vi "Get Protocol.vi"(8 "error in (no error)":errorcluster, 11 "instrument addon refnum in":T1 format="%.0x") -> (0 "error out":errorcluster, 2 "protocol":refnum<class "Protocol Parent.lvclass">, 3 "instrument addon refnum out":T1=18446744073709551615 format="%.0x")   [LabVIEW 2020, in "Instrument Addon Scripting API.lvlib"]
doc: "Outputs a protocol object based on the specified Instrument Addon Custom Device. \n\nThe protocol is formatted as one of the following classes: TCP.lvclass, UDP.lvclass, VISA.lvclass, RS-xxx.lvclass, AK TCP.lvclass, AK RS-xxx.lvclass, RS-xxx to GPIB ConvBox.lvclass"
uses:
  Instrument Addon Scripting API.lvlib
  <vilib>/NI VeriStand/Custom Device API/Custom Device Item Ref.ctl
  Includes/Protocols.lvlibp/Protocol Parent/Protocol Parent.lvclass
  Addon/Addon Shared/Types/FG Control.ctl
  Includes/Protocols.lvlibp/RS-xxx/RS-xxx.lvclass
  C:/Users/nitest/Desktop/Git 2020/niveristand-instrument-addon-custom-device/Includes/Protocols.lvlibp/Protocol Parent/Protocol Parent.lvclass
  Includes/Protocols.lvlibp/AK RS-xxx/AK RS-xxx.lvclass
  C:/Users/nitest/Desktop/Git 2020/niveristand-instrument-addon-custom-device/Includes/Protocols.lvlibp/RS-xxx/RS-xxx.lvclass
  Includes/Protocols.lvlibp/VISA/VISA.lvclass
  Includes/Protocols.lvlibp/AK TCP/AK TCP.lvclass
  C:/Users/nitest/Desktop/Git 2020/niveristand-instrument-addon-custom-device/Includes/Protocols.lvlibp/TCP/TCP.lvclass
  Includes/Protocols.lvlibp/TCP/TCP.lvclass
  Includes/Protocols.lvlibp/UDP/UDP.lvclass
  Includes/Protocols.lvlibp/RS-xxx to GPIB ConvBox/RS-xxx to GPIB ConvBox.lvclass
  Addon/Addon Shared/SubVIs/Constants.vi
  <vilib>/NI/NI VeriStand Advanced SysDef API/SysDef API/SysDef.Property.Get.vi
  <vilib>/NI/NI VeriStand Advanced SysDef API/_SubVIs/SysDef.Property.Get.String.vi
  <vilib>/NI/NI VeriStand Advanced SysDef API/SysDef API/SysDef.Property.Set.vi
  <vilib>/NI/NI VeriStand Advanced SysDef API/_SubVIs/SysDef.Property.Set.String.vi
  <vilib>/Utility/LVClass/Get LV Class Default Value.vi
  <vilib>/NI VeriStand/Custom Device API/NI VeriStand - Get Item Property.vi
  <vilib>/NI VeriStand/Custom Device API/Get Item Property (String).vi
  <vilib>/NI VeriStand/Custom Device API/Get Item Property (U32).vi
  <vilib>/NI VeriStand/Custom Device API/Get Item Property (Boolean).vi
  <vilib>/NI VeriStand/Custom Device API/NI VeriStand - Set Item Property.vi
  <vilib>/NI VeriStand/Custom Device API/Set Item Property (String).vi
  <vilib>/NI VeriStand/Custom Device API/Set Item Property (U32).vi
  <vilib>/NI VeriStand/Custom Device API/Set Item Property (Boolean).vi
  Includes/Protocols.lvlibp/RS-xxx/Data Access/Write PortSettings.vi
  Includes/Protocols.lvlibp/VISA/Data Access/Write VISA Resource.vi
  Includes/Protocols.lvlibp/VISA/Data Access/Write Enable Termination Character.vi
  Includes/Protocols.lvlibp/VISA/Data Access/Write Termination Character.vi
  Includes/Protocols.lvlibp/VISA/Data Access/Write Timeout.vi
  Includes/Protocols.lvlibp/VISA/Data Access/Write Append Write Termination Character.vi
  Includes/Protocols.lvlibp/TCP/Data Access/Write IP Address.vi
  Includes/Protocols.lvlibp/TCP/Data Access/Write Port.vi
  Includes/Protocols.lvlibp/UDP/Data Access/Write Local IP Address.vi
  Includes/Protocols.lvlibp/UDP/Data Access/Write Local Port.vi
  Includes/Protocols.lvlibp/UDP/Data Access/Write Target IP Address.vi
  Includes/Protocols.lvlibp/UDP/Data Access/Write Target Port.vi
  Includes/Protocols.lvlibp/RS-xxx to GPIB ConvBox/Data Access/Write Port.vi
  Includes/Protocols.lvlibp/RS-xxx to GPIB ConvBox/Data Access/Write ConvBox Address.vi
  Includes/Protocols.lvlibp/RS-xxx to GPIB ConvBox/Data Access/Write Assert Ren with IFC.vi
  Includes/Protocols.lvlibp/RS-xxx to GPIB ConvBox/Data Access/Write System controller.vi
  Includes/Protocols.lvlibp/RS-xxx to GPIB ConvBox/Data Access/Write IST bit sense.vi
  Includes/Protocols.lvlibp/RS-xxx to GPIB ConvBox/Data Access/Write GPIB Address.vi
  Addon/Addon Shared/Instrument Addon Shared.lvlib
  <vilib>/NI VeriStand/Custom Device API/Custom Device API.lvlib
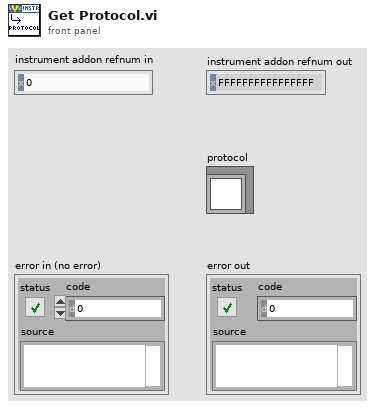
[diagram p1: front panel]
types:
  T1 = typedef "Custom Device API.lvlib/Custom Device Item Ref.ctl" = u64
  T2 = typedef "Instrument Addon Shared.lvlib/FG Control.ctl" = enum16{"Get", "Set"}
  T3 = cluster{"Port":string, "Baud Rate":u32, "Data Bits":u16, "Parity":enum16{"None", "Odd", "Even", "Mark", "Space"}, "Stop Bits":u16, "Flow Control":u16, "XON":enum16{"NUL", "SOH", "STX", "ETX", "EOT", "ENQ", "ACK", "BEL", "BS", "HT", "LF", "VT", "FF", "CR", "SO", "SI", "DLE", "DC1", "DC2", "DC3", "DC4", "NAK", "SYN", "ETB", "CAN", "EM", "SUB", "ESC", "FS", "GS", "RS", "US", "SP", "!", "\"", "#", "$", "%", "&", "'", "(", ")", "*", "+", ",", "- (-)", ".", "/", "0", "1", "2", "3", "4", "5", "6", "7", "8", "9", ":", ";", "<", "=", ">", "?", "@", "A", "B", "C", "D", "E", "F", "G", "H", "I", "J", "K", "L", "M", "N", "O", "P", "Q", "R", "S", "T", "U", "V", "W", "X", "Y", "Z", "[", "\\", "]", "^", "_", "`", "a", "b", "c", "d", "e", "f", "g", "h", "i", "j", "k", "l", "m", "n", "o", "p", "q", "r", "s", "t", "u", "v", "w", "x", "y", "z", "{", "|", "}", "~"}, "XOFF":enum16{"NUL", "SOH", "STX", "ETX", "EOT", "ENQ", "ACK", "BEL", "BS", "HT", "LF", "VT", "FF", "CR", "SO", "SI", "DLE", "DC1", "DC2", "DC3", "DC4", "NAK", "SYN", "ETB", "CAN", "EM", "SUB", "ESC", "FS", "GS", "RS", "US", "SP", "!", "\"", "#", "$", "%", "&", "'", "(", ")", "*", "+", ",", "- (-)", ".", "/", "0", "1", "2", "3", "4", "5", "6", "7", "8", "9", ":", ";", "<", "=", ">", "?", "@", "A", "B", "C", "D", "E", "F", "G", "H", "I", "J", "K", "L", "M", "N", "O", "P", "Q", "R", "S", "T", "U", "V", "W", "X", "Y", "Z", "[", "\\", "]", "^", "_", "`", "a", "b", "c", "d", "e", "f", "g", "h", "i", "j", "k", "l", "m", "n", "o", "p", "q", "r", "s", "t", "u", "v", "w", "x", "y", "z", "{", "|", "}", "~"}, "End Read on Termination Character":bool, "End Write on Termination Character":bool, "Termination Character":u8}
  T4 = typedef "Protocols.lvlibp/Protocol Parent.lvclass/Base Protocol Type.ctl" = enum16{"RS-XXX", "VISA", "TCPIP", "UDP", "GPIB ConvBox"}
  T5 = typedef "Instrument Addon Shared.lvlib/RSXXX Port Settings.ctl" = cluster{"Port":string, "Baud Rate":u32, "Data Bits":u16, "Parity":enum16{"None", "Odd", "Even", "Mark", "Space"}, "Stop Bits":u16, "Flow Control":u16, "XON":enum16{"NUL", "SOH", "STX", "ETX", "EOT", "ENQ", "ACK", "BEL", "BS", "HT", "LF", "VT", "FF", "CR", "SO", "SI", "DLE", "DC1", "DC2", "DC3", "DC4", "NAK", "SYN", "ETB", "CAN", "EM", "SUB", "ESC", "FS", "GS", "RS", "US", "SP", "!", "\"", "#", "$", "%", "&", "'", "(", ")", "*", "+", ",", "- (-)", ".", "/", "0", "1", "2", "3", "4", "5", "6", "7", "8", "9", ":", ";", "<", "=", ">", "?", "@", "A", "B", "C", "D", "E", "F", "G", "H", "I", "J", "K", "L", "M", "N", "O", "P", "Q", "R", "S", "T", "U", "V", "W", "X", "Y", "Z", "[", "\\", "]", "^", "_", "`", "a", "b", "c", "d", "e", "f", "g", "h", "i", "j", "k", "l", "m", "n", "o", "p", "q", "r", "s", "t", "u", "v", "w", "x", "y", "z", "{", "|", "}", "~"}, "XOFF":enum16{"NUL", "SOH", "STX", "ETX", "EOT", "ENQ", "ACK", "BEL", "BS", "HT", "LF", "VT", "FF", "CR", "SO", "SI", "DLE", "DC1", "DC2", "DC3", "DC4", "NAK", "SYN", "ETB", "CAN", "EM", "SUB", "ESC", "FS", "GS", "RS", "US", "SP", "!", "\"", "#", "$", "%", "&", "'", "(", ")", "*", "+", ",", "- (-)", ".", "/", "0", "1", "2", "3", "4", "5", "6", "7", "8", "9", ":", ";", "<", "=", ">", "?", "@", "A", "B", "C", "D", "E", "F", "G", "H", "I", "J", "K", "L", "M", "N", "O", "P", "Q", "R", "S", "T", "U", "V", "W", "X", "Y", "Z", "[", "\\", "]", "^", "_", "`", "a", "b", "c", "d", "e", "f", "g", "h", "i", "j", "k", "l", "m", "n", "o", "p", "q", "r", "s", "t", "u", "v", "w", "x", "y", "z", "{", "|", "}", "~"}, "End Read on Termination Character":bool, "End Write on Termination Character":bool, "Termination Character":u8}
  T6 = enum16{"NUL", "SOH", "STX", "ETX", "EOT", "ENQ", "ACK", "BEL", "BS", "HT", "LF", "VT", "FF", "CR", "SO", "SI", "DLE", "DC1", "DC2", "DC3", "DC4", "NAK", "SYN", "ETB", "CAN", "EM", "SUB", "ESC", "FS", "GS", "RS", "US", "SP", "!", "\"", "#", "$", "%", "&", "'", "(", ")", "*", "+", ",", "- (-)", ".", "/", "0", "1", "2", "3", "4", "5", "6", "7", "8", "9", ":", ";", "<", "=", ">", "?", "@", "A", "B", "C", "D", "E", "F", "G", "H", "I", "J", "K", "L", "M", "N", "O", "P", "Q", "R", "S", "T", "U", "V", "W", "X", "Y", "Z", "[", "\\", "]", "^", "_", "`", "a", "b", "c", "d", "e", "f", "g", "h", "i", "j", "k", "l", "m", "n", "o", "p", "q", "r", "s", "t", "u", "v", "w", "x", "y", "z", "{", "|", "}", "~"}
  T7 = typedef "Instrument Addon Shared.lvlib/VISA Settings.ctl" = cluster{"VISA Resource":string, "Enable Termination Character":bool, "Termination Character":u8, "Timeout":u32, "Append Write Termination Character":bool}
  T8 = typedef "Instrument Addon Shared.lvlib/TCPIP Settings.ctl" = cluster{"IP Address":string, "Port":u16}
  T9 = typedef "Instrument Addon Shared.lvlib/UDP Settings.ctl" = cluster{"Local IP Address":string, "Local Port":u16, "Target IP Address":string, "Target Port":u16}
  T10 = typedef "Instrument Addon Shared.lvlib/GPIB ConvBox Settings.ctl" = cluster{"Port":string, "ConvBox Address":string, "Assert Ren with IFC":bool, "System controller":bool, "IST bit sense":bool, "GPIB Address":string}
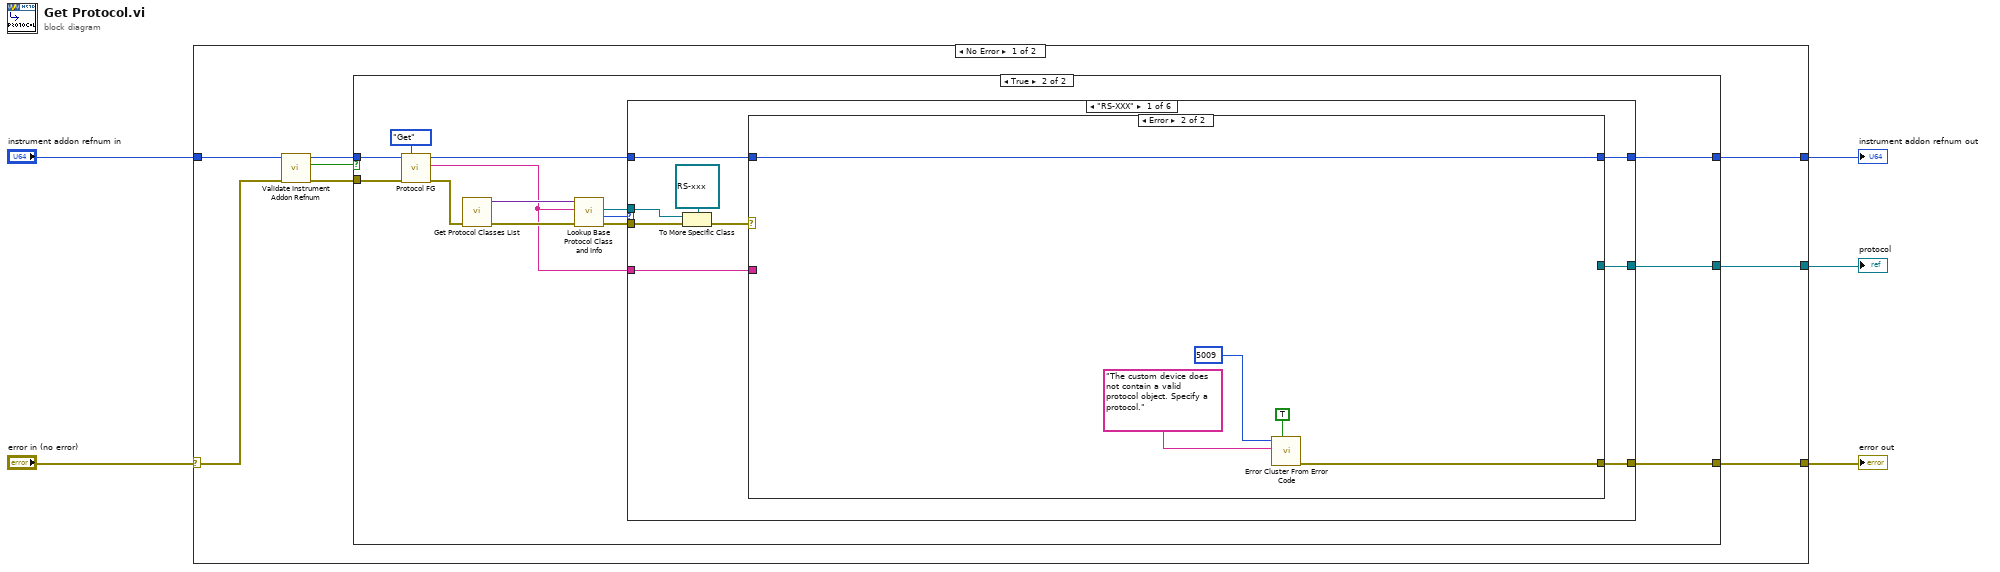
[diagram p0: block diagram]
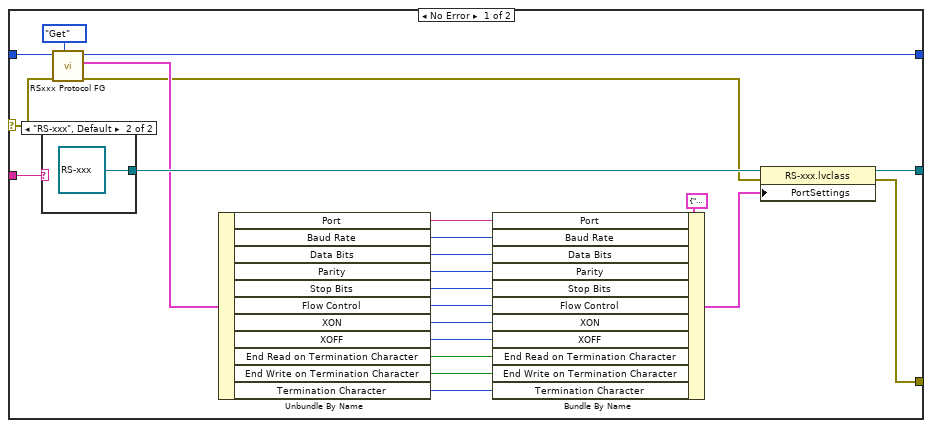
[diagram p3: hidden frame]
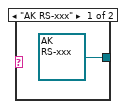
[diagram p4: hidden frame]
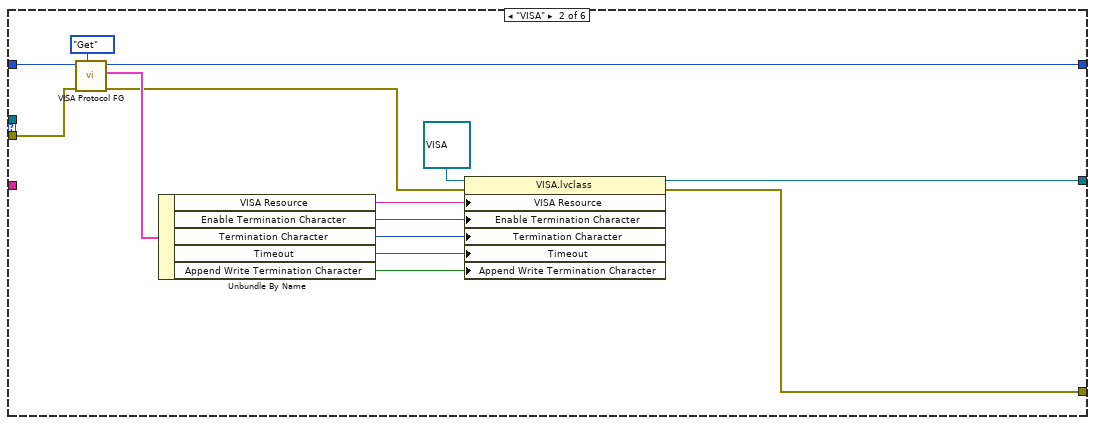
[diagram p5: hidden frame]
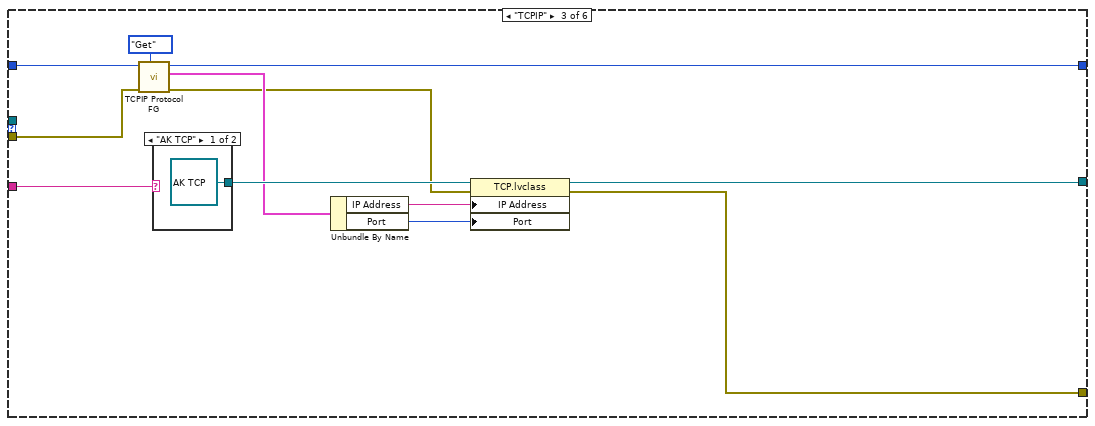
[diagram p6: hidden frame]
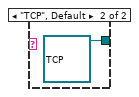
[diagram p7: hidden frame]
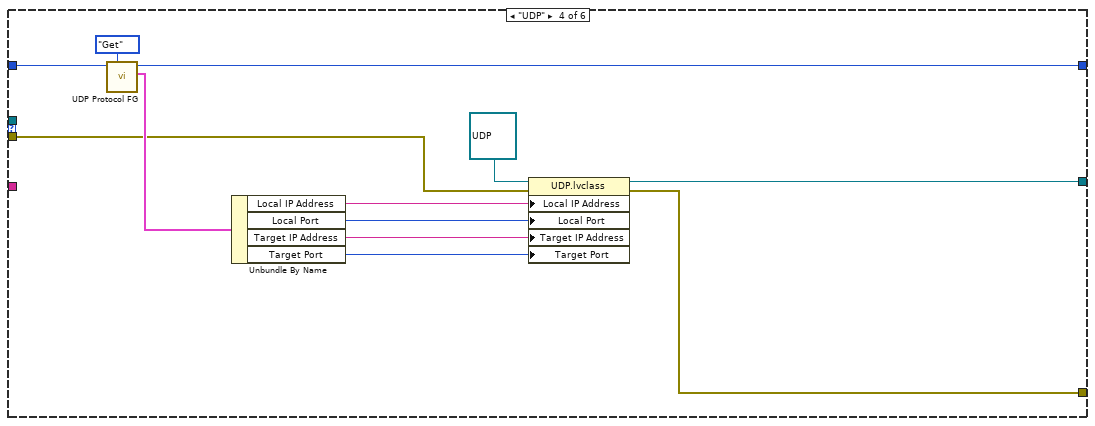
[diagram p8: hidden frame]
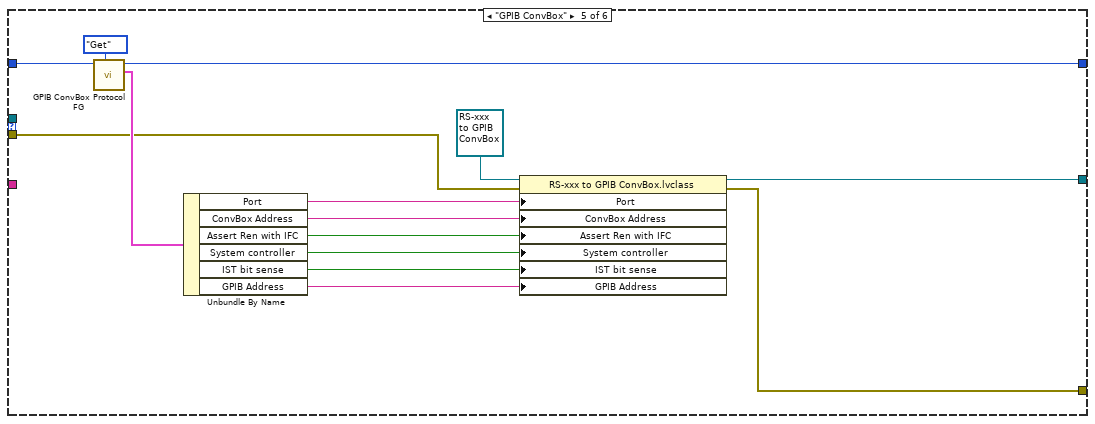
[diagram p9: hidden frame]
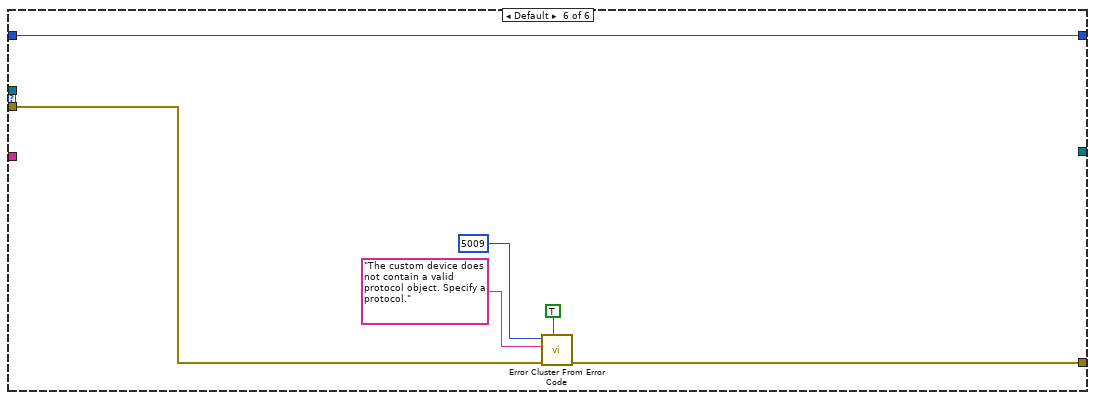
[diagram p10: hidden frame]
diagram:
  n1 = case shown="No Error" "error in (no error)" {
    selector: "error in (no error)" -> [w12 w130]
    tunnel: "instrument addon refnum in" -> [w13 w129]
    tunnel: [w9 w130] -> w4
    tunnel: [w8 w129] -> w2
    tunnel: [w6 _] -> w1
    frame No Error {
      n2 = call "Validate Instrument Addon Refnum.vi"("Error In"=w12, "Refnum In"=w13) -> ("Error Out"=w7:errorcluster, "Is Instrument Addon?"=w10:bool, "Refnum Out"=w11:T1)  [unwired: 7 in]
      n3 = case shown="True" w10 {
        tunnel: w11 -> [w15 w28]
        tunnel: [w14 w17] -> w9
        tunnel: [w15 w18] -> w8
        tunnel: w7 -> [w14 w27]
        tunnel: [_ w19] -> w6
        frame False {
        }
        frame True {
          n4 = call "Protocol FG.vi"("Action"=FG_Control."Get", "error in (no error)"=w27, "Device Item Ref in"=w28) -> ("error out"=w26:errorcluster, "Protocol out"=w16:string, "Item Ref out"=w23:T1)  [unwired: 6 in]
          n5 = call "Get Protocol Classes List.vi"("error in (no error)"=w26) -> ("error out"=w25:errorcluster, "Class Lookup"=w24:variant)  [unwired: 9 in]
          n6 = call "Lookup Base Protocol Class and Info.vi"("error in (no error)"=w25, "Protocol in"=w16, "Class Lookup"=w24) -> ("error out"=w21:errorcluster, "Protocol out"=w22:T4, "Protocol Parent out"=w20:refnum<class "Protocol Parent.lvclass">)  [unwired: 4 in, 2 out]
          n7 = case shown="\"RS-XXX\"" w22 {
            tunnel: w23 -> [w37 w81 w91 w106 w120 w128]
            tunnel: w21 -> [w32 w80 w90 w97 w110 w125]
            tunnel: w20 -> [w33 _ _ _ _ _]
            tunnel: [w35 w73 w85 w99 w111 _] -> w19
            tunnel: [w36 w70 w84 w100 w112 w128] -> w18
            tunnel: [w34 w69 w83 w98 w109 w124] -> w17
            tunnel: w16 -> [w38 _ w94 _ _ _]
            frame "RS-XXX" {
              n8 = To More Specific Class(target class=refnum<class "RS-xxx.lvclass"> refnum ("Protocols.lvlibp:RS-xxx.lvclass"), reference=w33, error in=w32) -> (error out=w31:errorcluster)  [unwired: 1 out]
              n9 = case shown="Error" w31 {
                selector: w31 -> [w39 _]
                tunnel: w38 -> [w61 _]
                tunnel: w37 -> [w59 w65]
                tunnel: [w43 w65] -> w36
                tunnel: [w42 _] -> w35
                tunnel: [w40 w66] -> w34
                frame No Error {
                  n10 = case shown="\"RS-xxx\", Default" w61 {
                    tunnel: [refnum<class "AK RS-xxx.lvclass"> refnum ("Protocols.lvlibp:AK RS-xxx.lvclass") refnum<class "RS-xxx.lvclass"> refnum ("Protocols.lvlibp:RS-xxx.lvclass")] -> w58
                    frame "AK RS-xxx" {
                    }
                    frame "RS-xxx", Default {
                    }
                  }
                  n11 = call "RSxxx Protocol FG.vi"("Action"=FG_Control."Get", "error in (no error)"=w39, "Device Item Ref in"=w59) -> ("error out"=w41:errorcluster, "Serial Config"=w56:T5, "Item Ref out"=w43:T1)  [unwired: 6 in]
                  n12 = Unbundle By Name(w56) -> ("Port"=w55:string, "Baud Rate"=w54:u32, "Data Bits"=w53:u16, "Parity"=w52:enum16{"None", "Odd", "Even", "Mark", "Space"}, "Stop Bits"=w51:u16, "Flow Control"=w50:u16, "XON"=w49:T6, "XOFF"=w48:T6, "End Read on Termination Character"=w47:bool, "End Write on Termination Character"=w46:bool, "Termination Character"=w45:u8)
                  n13 = Bundle By Name(cluster=T3 {"Port"="COM1", "Baud Rate"=9600, "Data Bits"=8, "Parity"=enum."None", "Stop Bits"=10, "Flow Control"=0, "XON"=enum."DC1", "XOFF"=enum."DC3", "End Read on Termination Character"=TRUE, "End Write on Termination Character"=TRUE, "Termination Character"=10} ("PortSettings"), "Port"=w55, "Baud Rate"=w54, "Data Bits"=w53, "Parity"=w52, "Stop Bits"=w51, "Flow Control"=w50, "XON"=w49, "XOFF"=w48, "End Read on Termination Character"=w47, "End Write on Termination Character"=w46, "Termination Character"=w45) -> (w44:T3)
                  n14 = property class="RS-xxx.lvclass"(reference=w58, error in=w41, "PortSettings"=w44) -> (reference out=w42:refnum<class "RS-xxx.lvclass">, error out=w40:errorcluster)
                }
                frame Error {
                  n15 = call <vilib>:"Error Cluster From Error Code.vi"("show call chain? (False)"=TRUE, "error message (\"\")"="The custom device does not contain a valid protocol object. Specify a protocol." ("error message (\"\")"), "error code (0)"=5009) -> ("error out"=w66:errorcluster)  [unwired: 6 in]
                }
              }
            }
            frame "VISA" {
              n16 = call "VISA Protocol FG.vi"("Action"=FG_Control."Get", "error in (no error)"=w80, "Device Item Ref in"=w81) -> ("error out"=w71:errorcluster, "VISA Config"=w79:T7, "Item Ref out"=w70:T1)  [unwired: 6 in]
              n17 = Unbundle By Name(w79) -> ("VISA Resource"=w78:string, "Enable Termination Character"=w77:bool, "Termination Character"=w76:u8, "Timeout"=w75:u32, "Append Write Termination Character"=w74:bool)
              n18 = property class="VISA.lvclass"(reference=refnum<class "VISA.lvclass"> refnum ("Protocols.lvlibp:VISA.lvclass"), error in=w71, "VISA Resource"=w78, "Enable Termination Character"=w77, "Termination Character"=w76, "Timeout"=w75, "Append Write Termination Character"=w74) -> (reference out=w73:refnum<class "VISA.lvclass">, error out=w69:errorcluster)
            }
            frame "TCPIP" {
              n19 = call "TCPIP Protocol FG.vi"("Action"=FG_Control."Get", "error in (no error)"=w90, "Device Item Ref in"=w91) -> ("error out"=w86:errorcluster, "TCP/IP Config"=w89:T8, "Item Ref out"=w84:T1)  [unwired: 6 in]
              n20 = case shown="\"AK TCP\"" w94 {
                tunnel: [refnum<class "AK TCP.lvclass"> refnum ("Protocols.lvlibp:AK TCP.lvclass") refnum<class "TCP.lvclass"> refnum ("Protocols.lvlibp:TCP.lvclass")] -> w93
                frame "AK TCP" {
                }
                frame "TCP", Default {
                }
              }
              n21 = Unbundle By Name(w89) -> ("IP Address"=w88:string, "Port"=w87:u16)
              n22 = property class="TCP.lvclass"(reference=w93, error in=w86, "IP Address"=w88, "Port"=w87) -> (reference out=w85:refnum<class "TCP.lvclass">, error out=w83:errorcluster)
            }
            frame "UDP" {
              n23 = call "UDP Protocol FG.vi"("Action"=FG_Control."Get", "Device Item Ref in"=w106) -> ("UDP Config"=w105:T9, "Item Ref out"=w100:T1)  [unwired: 7 in, 1 out]
              n24 = Unbundle By Name(w105) -> ("Local IP Address"=w104:string, "Local Port"=w103:u16, "Target IP Address"=w102:string, "Target Port"=w101:u16)
              n25 = property class="UDP.lvclass"(reference=refnum<class "UDP.lvclass"> refnum ("Protocols.lvlibp:UDP.lvclass"), error in=w97, "Local IP Address"=w104, "Local Port"=w103, "Target IP Address"=w102, "Target Port"=w101) -> (reference out=w99:refnum<class "UDP.lvclass">, error out=w98:errorcluster)
            }
            frame "GPIB ConvBox" {
              n26 = call "GPIB ConvBox Protocol FG.vi"("Action"=FG_Control."Get", "Device Item Ref in"=w120) -> ("GPIB ConvBox Config"=w119:T10, "Item Ref out"=w112:T1)  [unwired: 7 in, 1 out]
              n27 = Unbundle By Name(w119) -> ("Port"=w118:string, "ConvBox Address"=w117:string, "Assert Ren with IFC"=w116:bool, "System controller"=w115:bool, "IST bit sense"=w114:bool, "GPIB Address"=w113:string)
              n28 = property class="RS-xxx to GPIB ConvBox.lvclass"(reference=refnum<class "RS-xxx to GPIB ConvBox.lvclass"> refnum ("Protocols.lvlibp:RS-xxx to GPIB ConvBox.lvclass"), error in=w110, "Port"=w118, "ConvBox Address"=w117, "Assert Ren with IFC"=w116, "System controller"=w115, "IST bit sense"=w114, "GPIB Address"=w113) -> (reference out=w111:refnum<class "RS-xxx to GPIB ConvBox.lvclass">, error out=w109:errorcluster)
            }
            frame Default {
              n29 = call <vilib>:"Error Cluster From Error Code.vi"("show call chain? (False)"=TRUE, "error in (no error)"=w125, "error message (\"\")"="The custom device does not contain a valid protocol object. Specify a protocol." ("error message (\"\")"), "error code (0)"=5009) -> ("error out"=w124:errorcluster)  [unwired: 5 in]
            }
          }
        }
      }
    }
    frame Error {
    }
  }
  "error out" <- w4
  "instrument addon refnum out" <- w2
  "protocol" <- w1
